vi "main.vi"() -> ()   [LabVIEW 2014]
uses:
  controls/addressPF.ctl
  controls/dataPF.ctl
  <vilib>/rvi/interface/nirviReadWriteControl/nirviReadWriteControl.xnode
  NiFpgaLv.dll
  <vilib>/Utility/error.llb/Error Cluster From Error Code.vi
  <vilib>/rvi/interface/Simulation/niFpgaSimulationCallBeginRW.vi
  <vilib>/rvi/errors/niLvFpgaAdjustHostInterfaceError.vi
  <vilib>/rvi/interface/nirviOpenFPGA/nirviOpenFPGA.xnode
  <vilib>/rvi/Analysis/host/Public/NI_FpgaMspHost.lvlib
  <vilib>/rvi/interface/nirviMethod/nirviMethod.xnode
  <vilib>/rvi/errors/niLvFpgaMergeErrorWithErrorCode.vi
  <vilib>/FPGAPlugInAG/Dynamic/niLvFpga_StartFifo_Dynamic.vi
  <vilib>/FPGAPlugInAG/Dynamic/niLvFpga_ConfigureFifo_Dynamic.vi
  <vilib>/FPGAPlugInAG/Dynamic/niLvFpga_ReadFifo_Dynamic.vi
  <vilib>/FPGAPlugInAG/Dynamic/niLvFpga_StopFifo_Dynamic.vi
  <vilib>/rvi/interface/nirviCloseFPGA/nirviCloseFPGA.xnode
  <vilib>/FPGAPlugInAG/Dynamic/niLvFpga_Close_Dynamic.vi
  <vilib>/FPGAPlugInAG/Dynamic/niLvFpga_Run_Dynamic.vi
  <vilib>/rvi/Analysis/host/Private/Sample Rate To Loop Time (ticks).vi
  FPGA Bitfiles/projetofinal_FPGATarget_acquiringdata_+swI5PFvCiE.lvbitx
  acquiring data.vi
  <vilib>/FPGAPlugInAG/myRIO-1900/niLvFpga_Open_myRIO-1900.vi
  <vilib>/rvi/interface/common/dynamic/niFpgaDynamicAddResources.vi
  FPGA Bitfiles/projetofinal_FPGATarget_fpga6_P5NV++MLsEc.lvbitx
  fpga6.vi
panel:
  out "Voltage":dbl[](array[numeric])
  out "Current":dbl[](array[numeric])
  in  "curvas":string(combo)
  out "Standart Deviation":dbl
  out "Mean":dbl
  in  "file name":string="measure"
  out "source":string
  out "status":bool
  out "code":i32
  in  "measure":bool
  in  "Wait":u32
  in  "acq":bool
  in  "save":bool
  out "contdown":i16
  in  "duration":dbl=5.0 format="%#_13g"
  in  "f (Hz)":dbl=50000.0 format="%#_6p"
  in  "Stop Button":bool
  out "FIFO full?":bool
  in  "set":bool
  in  "qvolt":i32
  in  "sens":i32
  in  "bi":bool
  in  "qvolt":bool
  in  "sens":bool caption="sensibility"
  in  "mode":string(combo)
  # "Programming"
  # "Acquisition"
  # "Save File"
  # "Sensibility"
  # "File Name"
  # "Frequency (Hz)"
  # "Quiescent Voltage"
  # "FIFO Full"
  # "Unipolar"
  # "Duration"
  # "Countdown"
  # "Measure"
  # "Wait"
  # "Error"
  # "Status"
  # "Source"
  # "Code"
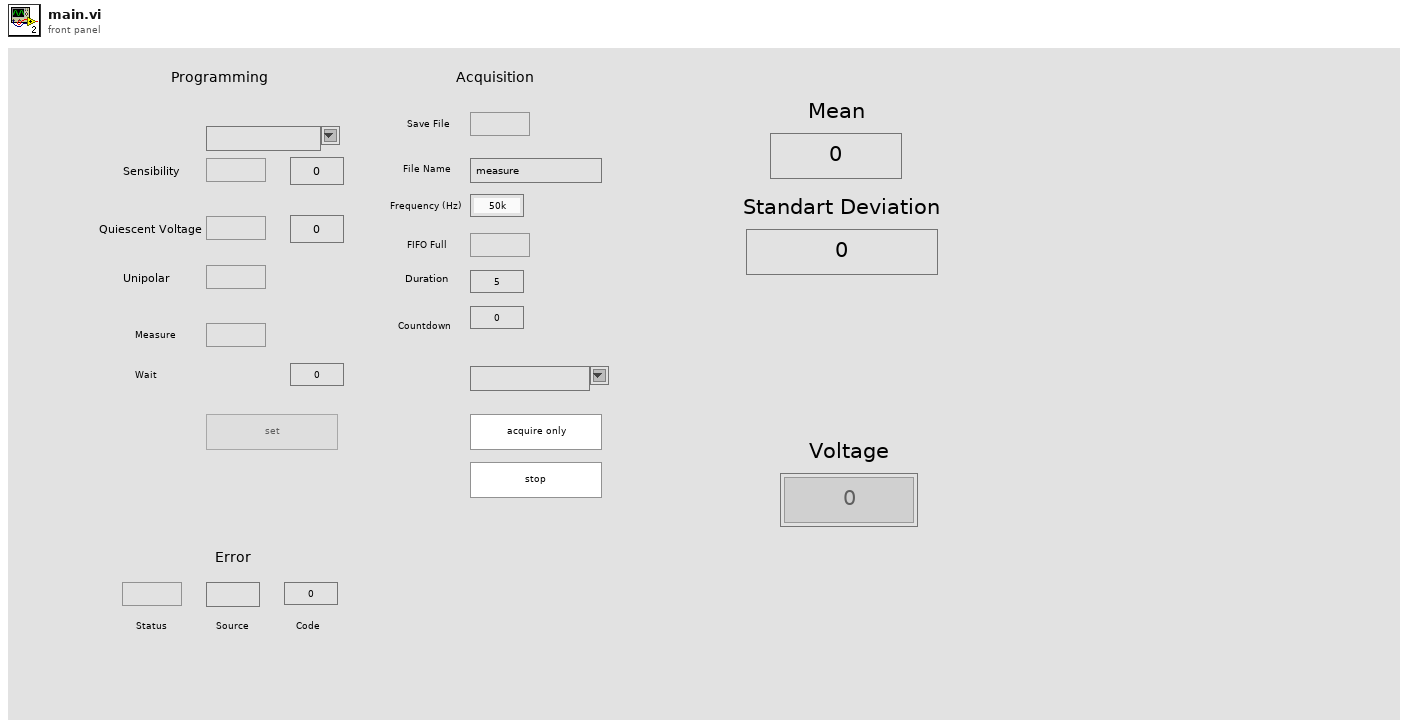
[diagram p1: front panel]
types:
  T1 = enum8{"Enabled", "Disabled", "Disabled and Grayed Out"}
  T2 = typedef "dataPF.ctl" = cluster{"sens":i32, "set?":bool, "mode":string, "parameters":cluster{"sens":bool, "qvolt":bool, "bi":bool}, "counter":i32, "qvolt":i32, "data":dbl[][], "fpga ref":refnum<k20>, "frequency":dbl}
  T3 = typedef "addressPF.ctl" = enum16{"idle", "lock", "set", "reset", "get data", "save data"}
  T4 = cluster{"mean":dbl, "standard deviation":dbl, "variance":dbl}
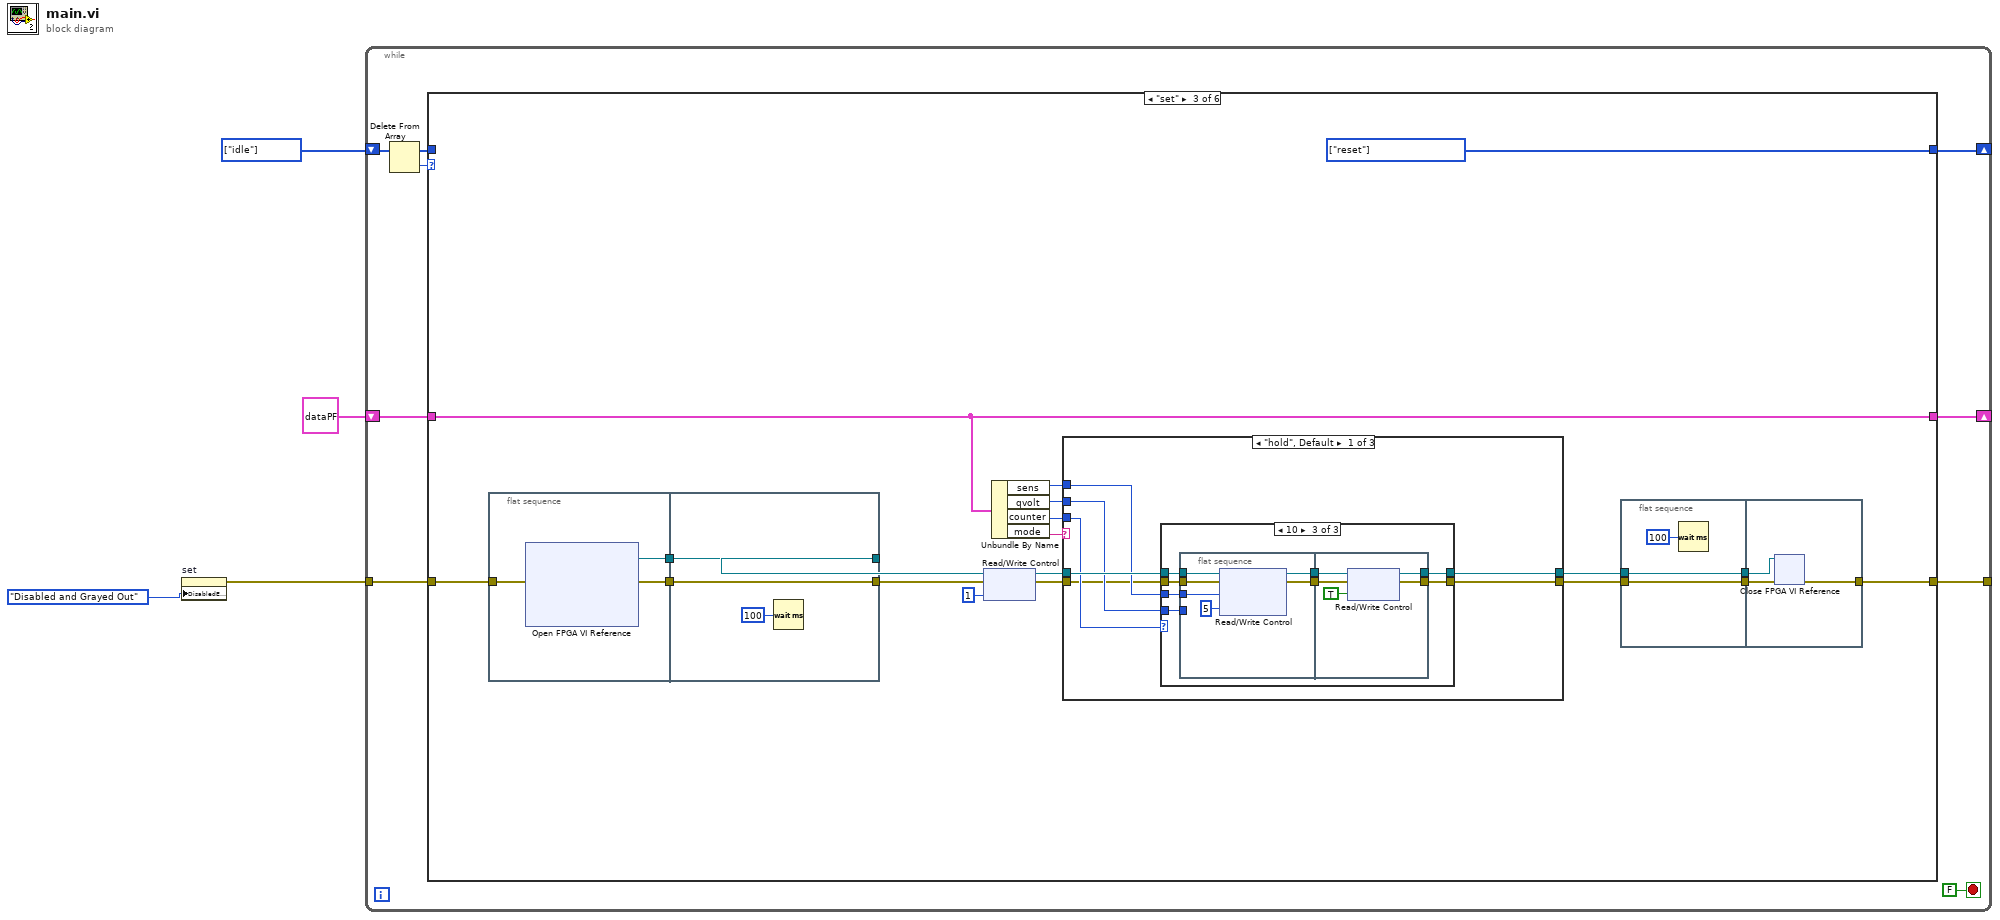
[diagram p0: block diagram]
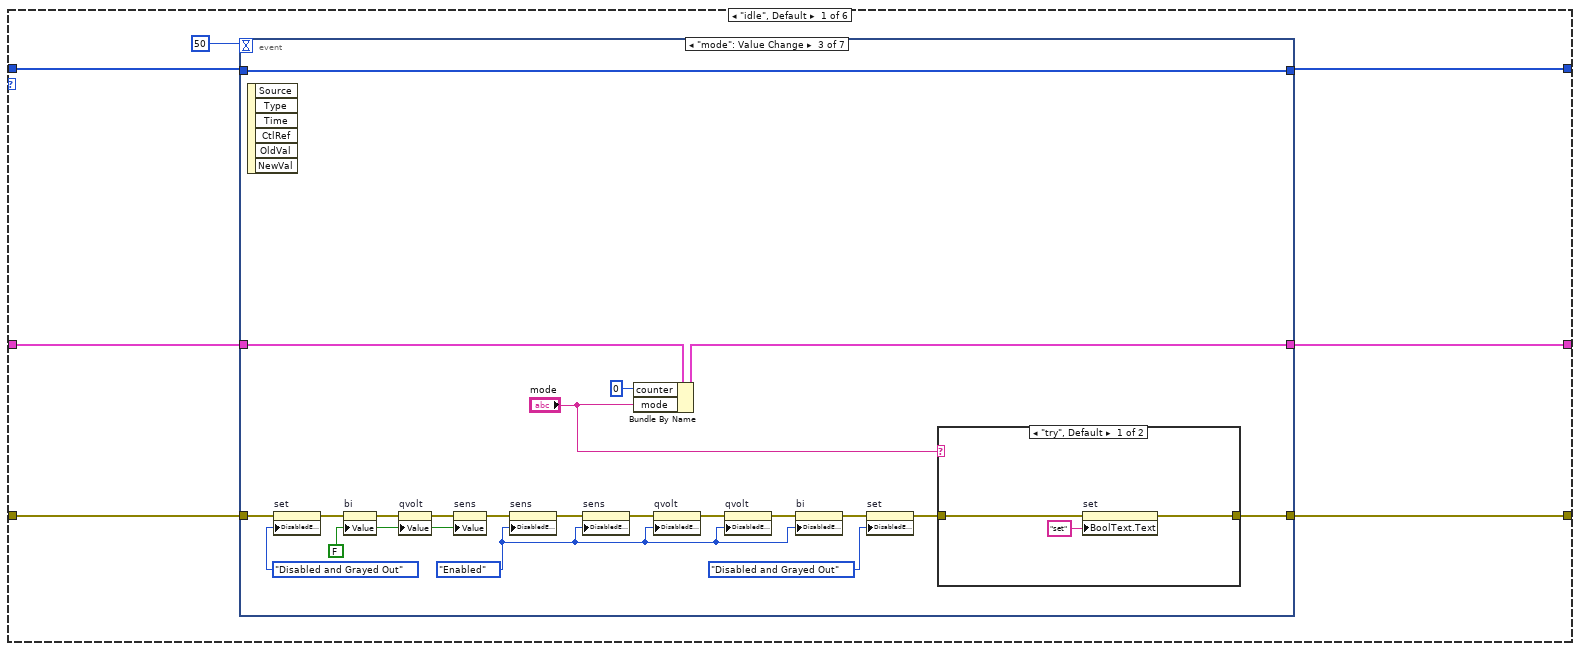
[diagram p2: hidden frame]
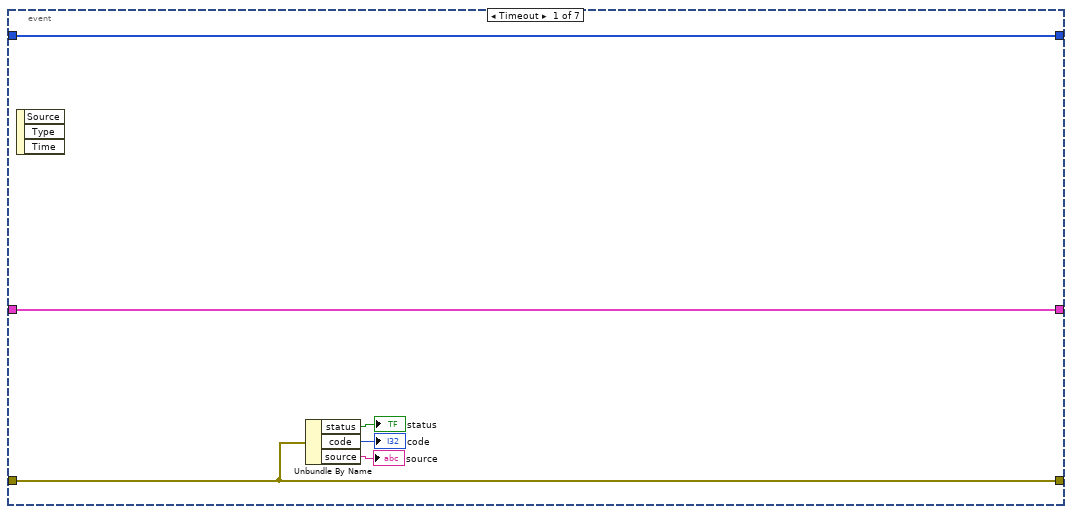
[diagram p3: hidden frame]
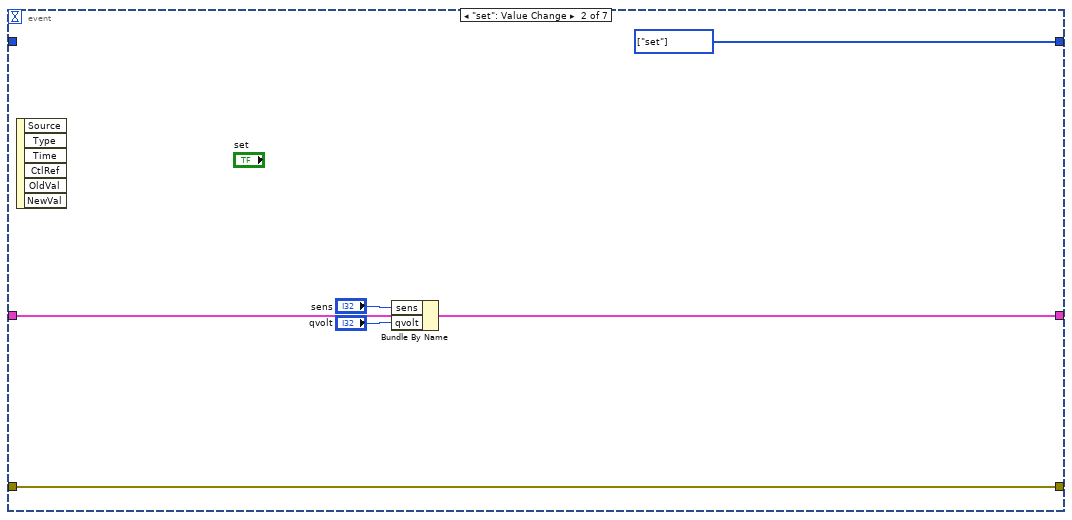
[diagram p4: hidden frame]
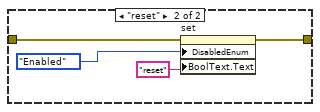
[diagram p5: hidden frame]
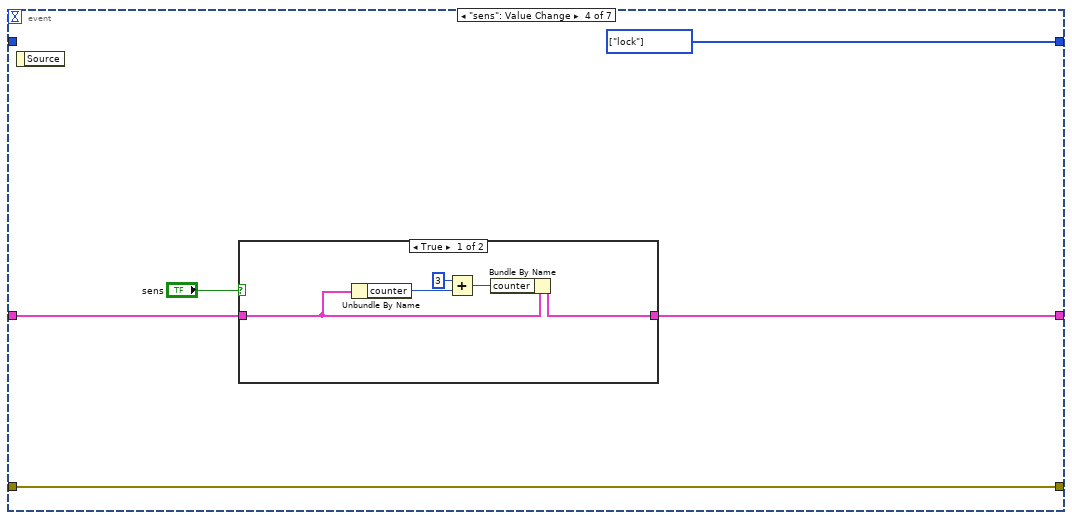
[diagram p6: hidden frame]
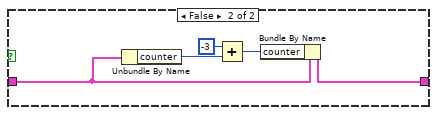
[diagram p7: hidden frame]
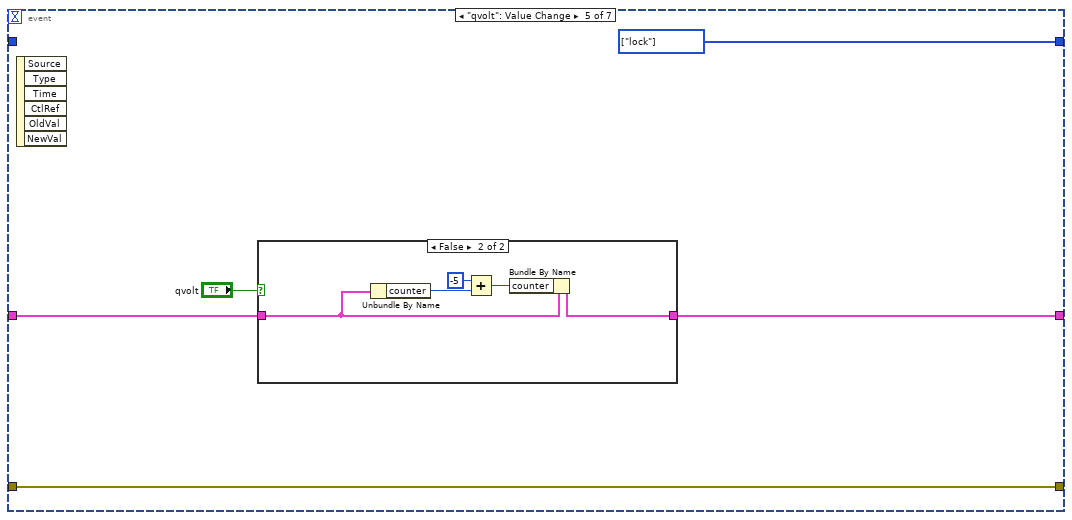
[diagram p8: hidden frame]
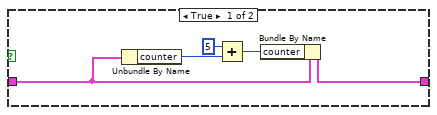
[diagram p9: hidden frame]
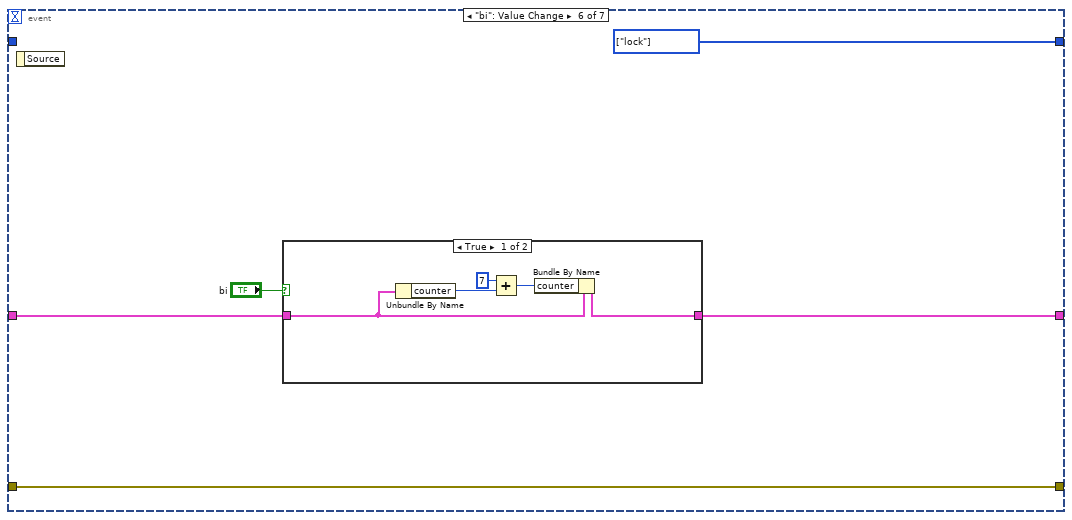
[diagram p10: hidden frame]
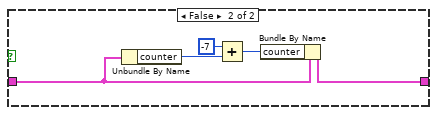
[diagram p11: hidden frame]
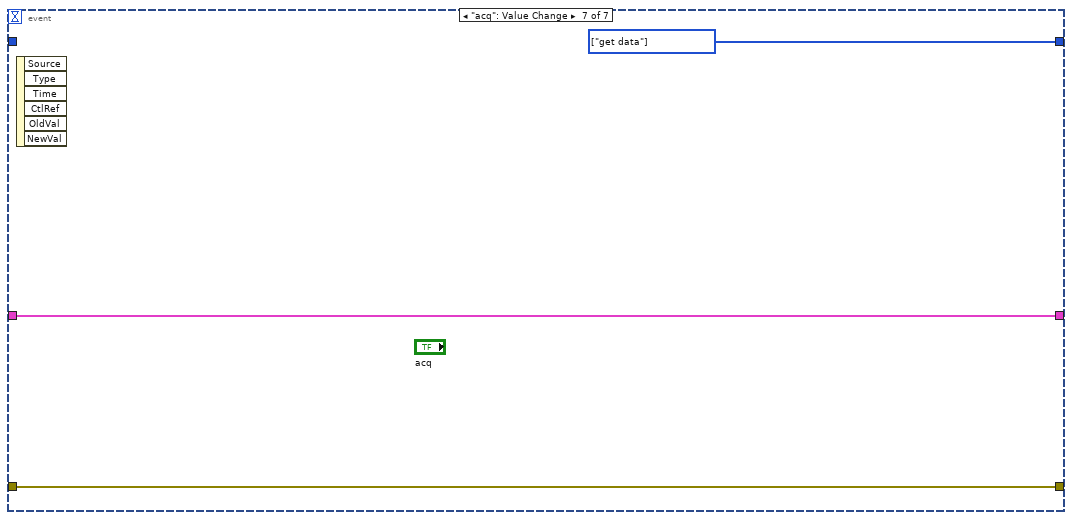
[diagram p12: hidden frame]
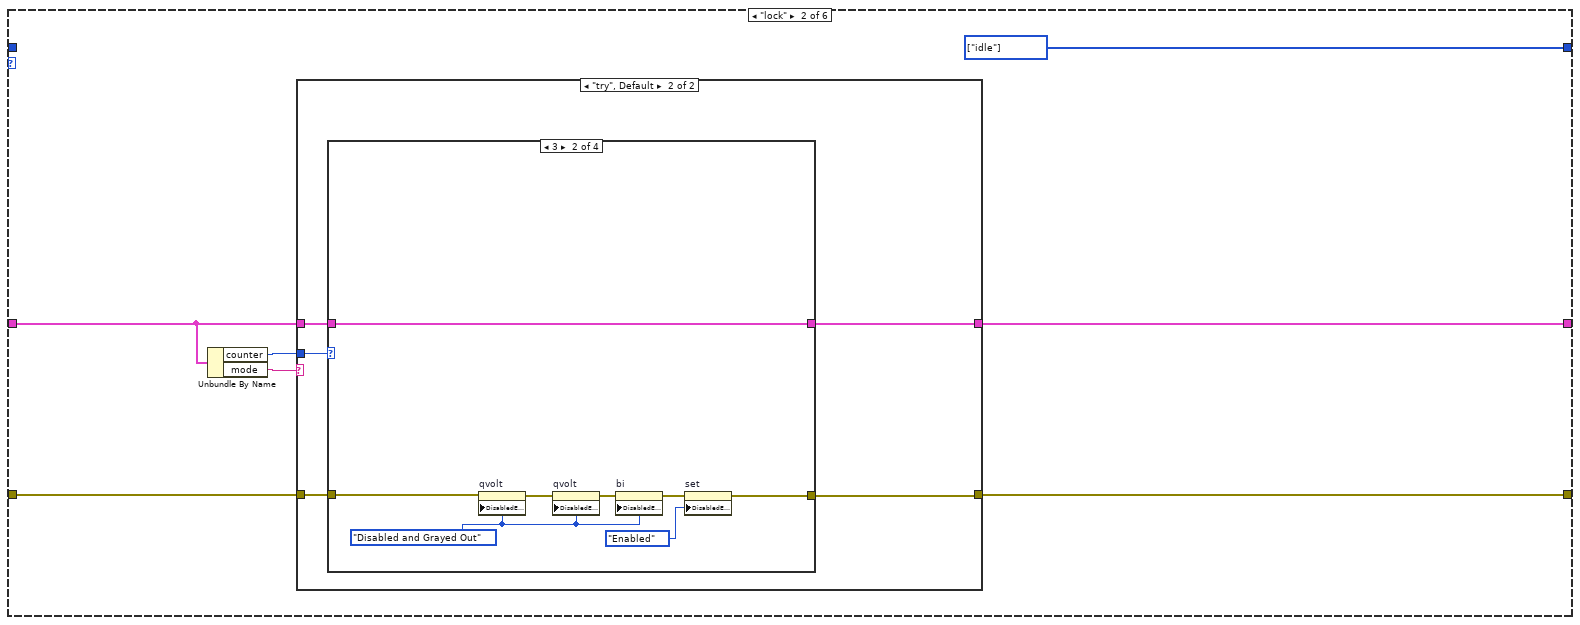
[diagram p13: hidden frame]
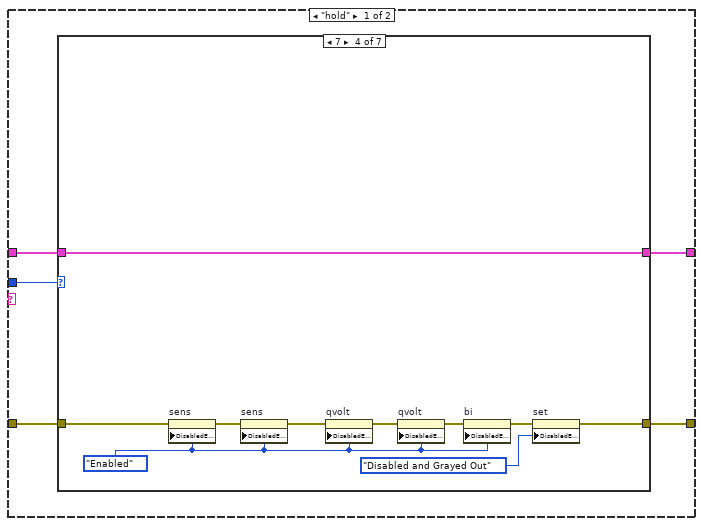
[diagram p14: hidden frame]
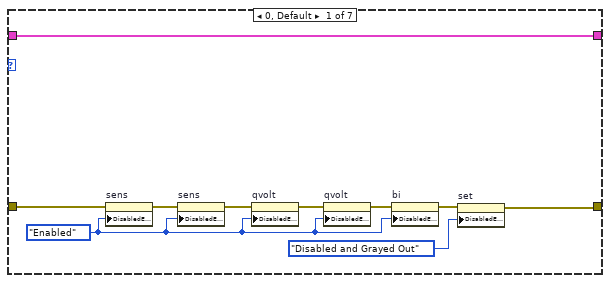
[diagram p15: hidden frame]
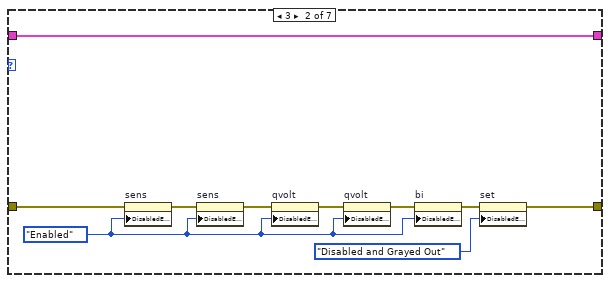
[diagram p16: hidden frame]
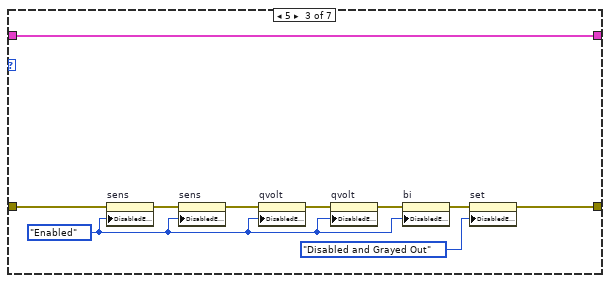
[diagram p17: hidden frame]
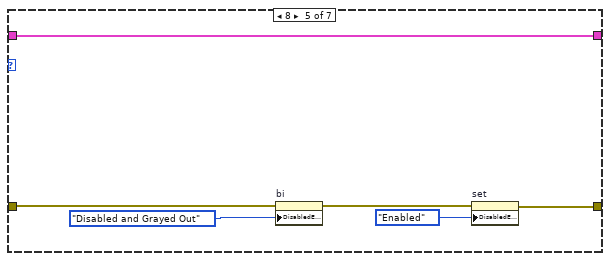
[diagram p18: hidden frame]
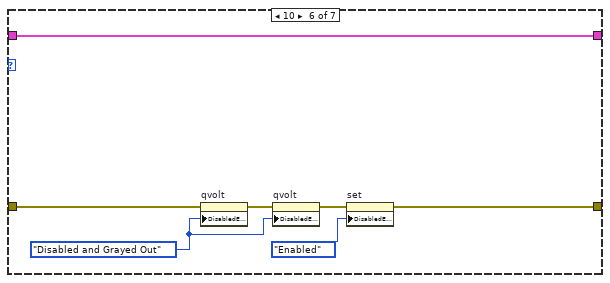
[diagram p19: hidden frame]
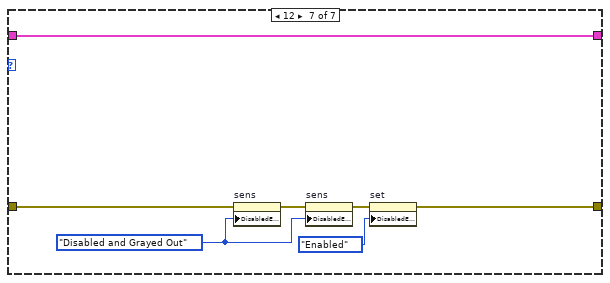
[diagram p20: hidden frame]
diagram:
  w4 = T3[] [enum."idle"] items=["idle", "lock", "set", "reset", "get data", "save data"]
  n1 = property on="set" class="Bool"("DisabledEnum"=T1."Disabled and Grayed Out" ("Disabled")) -> (error out=w1:errorcluster)  [unwired: 2 in, 1 out]
  n2 = while {
    shift-right: [w10] -> _
    shift-left: w4 -> [w13]
    shift-right: [w8] -> _
    shift-left: T2 {"sens"=0, "set?"=FALSE, "mode"="", "parameters"={"sens"=FALSE, "qvolt"=FALSE, "bi"=FALSE}, "counter"=0, "qvolt"=0, "data"=[], "fpga ref"=refnum, "frequency"=0.0} -> [w7]
    tunnel: w1 -> [w6]
    tunnel: [w5] -> _
    stop <- FALSE stop-if-true
    n3 = Delete From Array(array=w13) -> (deleted portion=w12:T3, array with subset deleted=w11:T3[])  [unwired: 2 in]
    n4 = case shown="\"set\"" w12 {
      tunnel: w11 -> [w20 _ _ _ _ _]
      tunnel: [w19 w115 w239 w384 w413 w493] -> w10
      tunnel: [w18 w112 w231 w386 w428 w492] -> w8
      tunnel: w7 -> [w17 w111 w231 w377 w430 w492]
      tunnel: w6 -> [w15 w110 w227 w380 w426 w485]
      tunnel: [w14 w109 w230 w385 w422 w490] -> w5
      frame "idle", Default {
        n5 = event shown="[2] \"mode\": Value Change" {
          selector: _ -> [_ _ _ _ _ _ _]
          dyn-events: _ -> [_ _ _ _ _ _ _]
          timeout: 50 -> [_ _ _ _ _ _ _]
          tunnel: w20 -> [w26 _ w53 _ _ _ _]
          tunnel: [w26 w32 w53 w65 w80 w95 w107] -> w19
          tunnel: [w25 w30 w51 w62 w79 w93 w106] -> w18
          tunnel: w17 -> [w25 w31 w52 w63 w78 w94 w106]
          tunnel: w15 -> [w24 w28 w37 w61 w76 w91 w108]
          tunnel: [w24 w28 w34 w61 w76 w91 w108] -> w14
          event Timeout {
            n6 = event-data() -> ()  [unwired: 1 in, 3 out]
            n7 = Unbundle By Name(w24) -> ("status"=→"status":bool, "code"=→"code":i32, "source"=→"source":string)
          }
          event "set": Value Change {
            w32 = T3[] [enum."set"] items=["idle", "lock", "set", "reset", "get data", "save data"]
            n8 = event-data() -> ()  [unwired: 1 in, 6 out]
            n9 = Bundle By Name(cluster=w31, "sens"="sens", "qvolt"="qvolt") -> (w30:T2)
          }
          event "mode": Value Change {
            w44 = T1."Enabled" ("Disabled")
            w50 = FALSE
            n10 = event-data() -> ()  [unwired: 1 in, 6 out]
            n11 = property on="set" class="Bool"(error in=w37, "DisabledEnum"=T1."Disabled and Grayed Out" ("Disabled")) -> (error out=w39:errorcluster)  [unwired: 1 in, 1 out]
            n12 = property on="bi" class="Bool (strict)"(error in=w39, "Value"=w50) -> (error out=w41:errorcluster)  [unwired: 1 in, 1 out]
            n13 = property on="qvolt" class="Bool (strict)"(error in=w41, "Value"=w50) -> (error out=w40:errorcluster)  [unwired: 1 in, 1 out]
            n14 = property on="sens" class="Bool (strict)"(error in=w40, "Value"=w50) -> (error out=w38:errorcluster)  [unwired: 1 in, 1 out]
            n15 = property on="sens" class="DigNum (strict)"(error in=w38, "DisabledEnum"=w44) -> (error out=w46:errorcluster)  [unwired: 1 in, 1 out]
            n16 = property on="sens" class="Bool (strict)"(error in=w46, "DisabledEnum"=w44) -> (error out=w36:errorcluster)  [unwired: 1 in, 1 out]
            n17 = Bundle By Name(cluster=w52, "counter"=0, "mode"="mode") -> (w51:T2)
            n18 = property on="qvolt" class="DigNum (strict)"(error in=w36, "DisabledEnum"=w44) -> (error out=w47:errorcluster)  [unwired: 1 in, 1 out]
            n19 = property on="qvolt" class="Bool (strict)"(error in=w47, "DisabledEnum"=w44) -> (error out=w48:errorcluster)  [unwired: 1 in, 1 out]
            n20 = property on="bi" class="Bool (strict)"(error in=w48, "DisabledEnum"=w44) -> (error out=w45:errorcluster)  [unwired: 1 in, 1 out]
            n21 = property on="set" class="Bool"(error in=w45, "DisabledEnum"=T1."Disabled and Grayed Out" ("Disabled")) -> (error out=w35:errorcluster)  [unwired: 1 in, 1 out]
            n22 = case shown="\"try\", Default" "mode" {
              tunnel: w35 -> [w56 w59]
              tunnel: [w55 w58] -> w34
              frame "try", Default {
                n23 = property on="set" class="Bool"(error in=w56, "BoolText.Text"="set" ("Boolean Text.Text")) -> (error out=w55:errorcluster)  [unwired: 1 in, 1 out]
              }
              frame "reset" {
                n24 = property on="set" class="Bool"(error in=w59, "DisabledEnum"=T1."Enabled" ("Disabled"), "BoolText.Text"="reset" ("Boolean Text.Text")) -> (error out=w58:errorcluster)  [unwired: 1 in, 1 out]
              }
            }
          }
          event "sens": Value Change {
            w65 = T3[] [enum."lock"] items=["idle", "lock", "set", "reset", "get data", "save data"]
            n25 = event-data() -> ()  [unwired: 1 in, 1 out]
            n26 = case shown="True" "sens" {
              tunnel: w63 -> [w67 w72]
              tunnel: [w66 w71] -> w62
              frame True {
                n27 = Unbundle By Name(w67) -> ("counter"=w69:i32)
                n28 = Add(x=3, y=w69) -> (x+y=w68:i32)
                n29 = Bundle By Name(cluster=w67, "counter"=w68) -> (w66:T2)
              }
              frame False {
                n30 = Unbundle By Name(w72) -> ("counter"=w74:i32)
                n31 = Add(x=-3, y=w74) -> (x+y=w73:i32)
                n32 = Bundle By Name(cluster=w72, "counter"=w73) -> (w71:T2)
              }
            }
          }
          event "qvolt": Value Change {
            w80 = T3[] [enum."lock"] items=["idle", "lock", "set", "reset", "get data", "save data"]
            n33 = event-data() -> ()  [unwired: 1 in, 6 out]
            n34 = case shown="False" "qvolt" {
              tunnel: w78 -> [w82 w87]
              tunnel: [w81 w86] -> w79
              frame True {
                n35 = Unbundle By Name(w82) -> ("counter"=w84:i32)
                n36 = Add(x=5, y=w84) -> (x+y=w83:i32)
                n37 = Bundle By Name(cluster=w82, "counter"=w83) -> (w81:T2)
              }
              frame False {
                n38 = Unbundle By Name(w87) -> ("counter"=w89:i32)
                n39 = Add(x=-5, y=w89) -> (x+y=w88:i32)
                n40 = Bundle By Name(cluster=w87, "counter"=w88) -> (w86:T2)
              }
            }
          }
          event "bi": Value Change {
            w95 = T3[] [enum."lock"] items=["idle", "lock", "set", "reset", "get data", "save data"]
            n41 = event-data() -> ()  [unwired: 1 in, 1 out]
            n42 = case shown="True" "bi" {
              tunnel: w94 -> [w97 w102]
              tunnel: [w96 w101] -> w93
              frame True {
                n43 = Unbundle By Name(w97) -> ("counter"=w99:i32)
                n44 = Add(x=7, y=w99) -> (x+y=w98:i32)
                n45 = Bundle By Name(cluster=w97, "counter"=w98) -> (w96:T2)
              }
              frame False {
                n46 = Unbundle By Name(w102) -> ("counter"=w104:i32)
                n47 = Add(x=-7, y=w104) -> (x+y=w103:i32)
                n48 = Bundle By Name(cluster=w102, "counter"=w103) -> (w101:T2)
              }
            }
          }
          event "acq": Value Change {
            w107 = T3[] [enum."get data"] items=["idle", "lock", "set", "reset", "get data", "save data"]
            n49 = event-data() -> ()  [unwired: 1 in, 6 out]
          }
        }
      }
      frame "lock" {
        w115 = T3[] [enum."idle"] items=["idle", "lock", "set", "reset", "get data", "save data"]
        n50 = Unbundle By Name(w111) -> ("counter"=w113:i32, "mode"=w114:string)
        n51 = case shown="\"try\", Default" w114 {
          tunnel: w113 -> [w120 w185]
          tunnel: [w116 w182] -> w112
          tunnel: w111 -> [w117 w181]
          tunnel: w110 -> [w119 w184]
          tunnel: [w118 w183] -> w109
          frame "hold" {
            n52 = case shown="7" w120 {
              tunnel: w119 -> [w124 w132 w144 w152 w162 w169 w176]
              tunnel: [w122 w133 w143 w153 w164 w168 w174] -> w118
              tunnel: w117 -> [w121 w131 w141 w151 w161 w167 w177]
              tunnel: [w121 w131 w141 w151 w161 w167 w177] -> w116
              frame 0, Default {
                w126 = T1."Enabled" ("Disabled")
                n53 = property on="sens" class="DigNum (strict)"(error in=w124, "DisabledEnum"=w126) -> (error out=w127:errorcluster)  [unwired: 1 in, 1 out]
                n54 = property on="sens" class="Bool (strict)"(error in=w127, "DisabledEnum"=w126) -> (error out=w128:errorcluster)  [unwired: 1 in, 1 out]
                n55 = property on="qvolt" class="DigNum (strict)"(error in=w128, "DisabledEnum"=w126) -> (error out=w129:errorcluster)  [unwired: 1 in, 1 out]
                n56 = property on="qvolt" class="Bool (strict)"(error in=w129, "DisabledEnum"=w126) -> (error out=w130:errorcluster)  [unwired: 1 in, 1 out]
                n57 = property on="bi" class="Bool (strict)"(error in=w130, "DisabledEnum"=w126) -> (error out=w123:errorcluster)  [unwired: 1 in, 1 out]
                n58 = property on="set" class="Bool"(error in=w123, "DisabledEnum"=T1."Disabled and Grayed Out" ("Disabled")) -> (error out=w122:errorcluster)  [unwired: 1 in, 1 out]
              }
              frame 3 {
                w136 = T1."Enabled" ("Disabled")
                n59 = property on="sens" class="DigNum (strict)"(error in=w132, "DisabledEnum"=w136) -> (error out=w137:errorcluster)  [unwired: 1 in, 1 out]
                n60 = property on="sens" class="Bool (strict)"(error in=w137, "DisabledEnum"=w136) -> (error out=w138:errorcluster)  [unwired: 1 in, 1 out]
                n61 = property on="qvolt" class="DigNum (strict)"(error in=w138, "DisabledEnum"=w136) -> (error out=w139:errorcluster)  [unwired: 1 in, 1 out]
                n62 = property on="qvolt" class="Bool (strict)"(error in=w139, "DisabledEnum"=w136) -> (error out=w140:errorcluster)  [unwired: 1 in, 1 out]
                n63 = property on="bi" class="Bool (strict)"(error in=w140, "DisabledEnum"=w136) -> (error out=w134:errorcluster)  [unwired: 1 in, 1 out]
                n64 = property on="set" class="Bool"(error in=w134, "DisabledEnum"=T1."Disabled and Grayed Out" ("Disabled")) -> (error out=w133:errorcluster)  [unwired: 1 in, 1 out]
              }
              frame 5 {
                w142 = T1."Enabled" ("Disabled")
                n65 = property on="sens" class="DigNum (strict)"(error in=w144, "DisabledEnum"=w142) -> (error out=w147:errorcluster)  [unwired: 1 in, 1 out]
                n66 = property on="sens" class="Bool (strict)"(error in=w147, "DisabledEnum"=w142) -> (error out=w148:errorcluster)  [unwired: 1 in, 1 out]
                n67 = property on="qvolt" class="DigNum (strict)"(error in=w148, "DisabledEnum"=w142) -> (error out=w149:errorcluster)  [unwired: 1 in, 1 out]
                n68 = property on="qvolt" class="Bool (strict)"(error in=w149, "DisabledEnum"=w142) -> (error out=w150:errorcluster)  [unwired: 1 in, 1 out]
                n69 = property on="bi" class="Bool (strict)"(error in=w150, "DisabledEnum"=w142) -> (error out=w145:errorcluster)  [unwired: 1 in, 1 out]
                n70 = property on="set" class="Bool"(error in=w145, "DisabledEnum"=T1."Disabled and Grayed Out" ("Disabled")) -> (error out=w143:errorcluster)  [unwired: 1 in, 1 out]
              }
              frame 7 {
                w156 = T1."Enabled" ("Disabled")
                n71 = property on="sens" class="DigNum (strict)"(error in=w152, "DisabledEnum"=w156) -> (error out=w157:errorcluster)  [unwired: 1 in, 1 out]
                n72 = property on="sens" class="Bool (strict)"(error in=w157, "DisabledEnum"=w156) -> (error out=w158:errorcluster)  [unwired: 1 in, 1 out]
                n73 = property on="qvolt" class="DigNum (strict)"(error in=w158, "DisabledEnum"=w156) -> (error out=w159:errorcluster)  [unwired: 1 in, 1 out]
                n74 = property on="qvolt" class="Bool (strict)"(error in=w159, "DisabledEnum"=w156) -> (error out=w160:errorcluster)  [unwired: 1 in, 1 out]
                n75 = property on="bi" class="Bool (strict)"(error in=w160, "DisabledEnum"=w156) -> (error out=w154:errorcluster)  [unwired: 1 in, 1 out]
                n76 = property on="set" class="Bool"(error in=w154, "DisabledEnum"=T1."Disabled and Grayed Out" ("Disabled")) -> (error out=w153:errorcluster)  [unwired: 1 in, 1 out]
              }
              frame 8 {
                n77 = property on="bi" class="Bool (strict)"(error in=w162, "DisabledEnum"=T1."Disabled and Grayed Out" ("Disabled")) -> (error out=w163:errorcluster)  [unwired: 1 in, 1 out]
                n78 = property on="set" class="Bool"(error in=w163, "DisabledEnum"=T1."Enabled" ("Disabled")) -> (error out=w164:errorcluster)  [unwired: 1 in, 1 out]
              }
              frame 10 {
                w172 = T1."Disabled and Grayed Out" ("Disabled")
                n79 = property on="qvolt" class="DigNum (strict)"(error in=w169, "DisabledEnum"=w172) -> (error out=w173:errorcluster)  [unwired: 1 in, 1 out]
                n80 = property on="qvolt" class="Bool (strict)"(error in=w173, "DisabledEnum"=w172) -> (error out=w170:errorcluster)  [unwired: 1 in, 1 out]
                n81 = property on="set" class="Bool"(error in=w170, "DisabledEnum"=T1."Enabled" ("Disabled")) -> (error out=w168:errorcluster)  [unwired: 1 in, 1 out]
              }
              frame 12 {
                w179 = T1."Disabled and Grayed Out" ("Disabled")
                n82 = property on="sens" class="DigNum (strict)"(error in=w176, "DisabledEnum"=w179) -> (error out=w180:errorcluster)  [unwired: 1 in, 1 out]
                n83 = property on="sens" class="Bool (strict)"(error in=w180, "DisabledEnum"=w179) -> (error out=w175:errorcluster)  [unwired: 1 in, 1 out]
                n84 = property on="set" class="Bool"(error in=w175, "DisabledEnum"=T1."Enabled" ("Disabled")) -> (error out=w174:errorcluster)  [unwired: 1 in, 1 out]
              }
            }
          }
          frame "try", Default {
            n85 = case shown="3" w185 {
              tunnel: w184 -> [w187 w199 w205 w213]
              tunnel: [w188 w198 w206 w214] -> w183
              tunnel: [w186 w196 w204 w212] -> w182
              tunnel: w181 -> [w186 w196 w204 w212]
              frame 0, Default {
                w190 = T1."Enabled" ("Disabled")
                n86 = property on="sens" class="DigNum (strict)"(error in=w187, "DisabledEnum"=w190) -> (error out=w192:errorcluster)  [unwired: 1 in, 1 out]
                n87 = property on="sens" class="Bool (strict)"(error in=w192, "DisabledEnum"=w190) -> (error out=w193:errorcluster)  [unwired: 1 in, 1 out]
                n88 = property on="qvolt" class="DigNum (strict)"(error in=w193, "DisabledEnum"=w190) -> (error out=w194:errorcluster)  [unwired: 1 in, 1 out]
                n89 = property on="qvolt" class="Bool (strict)"(error in=w194, "DisabledEnum"=w190) -> (error out=w195:errorcluster)  [unwired: 1 in, 1 out]
                n90 = property on="bi" class="Bool (strict)"(error in=w195, "DisabledEnum"=w190) -> (error out=w191:errorcluster)  [unwired: 1 in, 1 out]
                n91 = property on="set" class="Bool"(error in=w191, "DisabledEnum"=T1."Disabled and Grayed Out" ("Disabled")) -> (error out=w188:errorcluster)  [unwired: 1 in, 1 out]
              }
              frame 3 {
                w197 = T1."Disabled and Grayed Out" ("Disabled")
                n92 = property on="qvolt" class="DigNum (strict)"(error in=w199, "DisabledEnum"=w197) -> (error out=w202:errorcluster)  [unwired: 1 in, 1 out]
                n93 = property on="qvolt" class="Bool (strict)"(error in=w202, "DisabledEnum"=w197) -> (error out=w203:errorcluster)  [unwired: 1 in, 1 out]
                n94 = property on="bi" class="Bool (strict)"(error in=w203, "DisabledEnum"=w197) -> (error out=w201:errorcluster)  [unwired: 1 in, 1 out]
                n95 = property on="set" class="Bool"(error in=w201, "DisabledEnum"=T1."Enabled" ("Disabled")) -> (error out=w198:errorcluster)  [unwired: 1 in, 1 out]
              }
              frame 5 {
                w210 = T1."Disabled and Grayed Out" ("Disabled")
                n96 = property on="sens" class="DigNum (strict)"(error in=w205, "DisabledEnum"=w210) -> (error out=w211:errorcluster)  [unwired: 1 in, 1 out]
                n97 = property on="sens" class="Bool (strict)"(error in=w211, "DisabledEnum"=w210) -> (error out=w209:errorcluster)  [unwired: 1 in, 1 out]
                n98 = property on="bi" class="Bool (strict)"(error in=w209, "DisabledEnum"=w210) -> (error out=w208:errorcluster)  [unwired: 1 in, 1 out]
                n99 = property on="set" class="Bool"(error in=w208, "DisabledEnum"=T1."Enabled" ("Disabled")) -> (error out=w206:errorcluster)  [unwired: 1 in, 1 out]
              }
              frame 7 {
                w218 = T1."Disabled and Grayed Out" ("Disabled")
                n100 = property on="sens" class="DigNum (strict)"(error in=w213, "DisabledEnum"=w218) -> (error out=w219:errorcluster)  [unwired: 1 in, 1 out]
                n101 = property on="sens" class="Bool (strict)"(error in=w219, "DisabledEnum"=w218) -> (error out=w217:errorcluster)  [unwired: 1 in, 1 out]
                n102 = property on="qvolt" class="DigNum (strict)"(error in=w217, "DisabledEnum"=w218) -> (error out=w220:errorcluster)  [unwired: 1 in, 1 out]
                n103 = property on="qvolt" class="Bool (strict)"(error in=w220, "DisabledEnum"=w218) -> (error out=w216:errorcluster)  [unwired: 1 in, 1 out]
                n104 = property on="set" class="Bool"(error in=w216, "DisabledEnum"=T1."Enabled" ("Disabled")) -> (error out=w214:errorcluster)  [unwired: 1 in, 1 out]
              }
            }
          }
        }
      }
      frame "set" {
        w239 = T3[] [enum."reset"] items=["idle", "lock", "set", "reset", "get data", "save data"]
        n105 = flat-sequence {
          tunnel: w227 -> [w242]
          tunnel: [w241] -> w222
          tunnel: [w240] -> w221
          tunnel: [w244] -> w225
          tunnel: [w245] -> w226
          tunnel: w222 -> [w245]
          tunnel: w221 -> [w244]
          frame #0 {
            n106 = xnode "Open FPGA VI Reference"("error in"=w242) -> ("FPGA VI Reference Out"=w240:refnum<k20>, "error out"=w241:errorcluster)  [unwired: 1 in]
          }
          frame #1 {
            n107 = Wait (ms)(milliseconds to wait=u32 100) -> ()  [unwired: 1 out]
          }
        }
        n108 = xnode "Read/Write Control"("FPGA VI Reference In"=w225, "error in"=w226, "treset"=u32 1) -> ("FPGA VI Reference Out"=w234:refnum<k20>, "error out"=w232:errorcluster)
        n109 = Unbundle By Name(w231) -> ("sens"=w236:i32, "qvolt"=w235:i32, "counter"=w237:i32, "mode"=w238:string)
        n110 = case shown="\"hold\", Default" w238 {
          tunnel: w237 -> [w257 _ w322]
          tunnel: w234 -> [w258 w303 w321]
          tunnel: w236 -> [w256 _ w320]
          tunnel: w235 -> [w255 _ w319]
          tunnel: [w254 w301 w318] -> w228
          tunnel: [w253 w300 w316] -> w229
          tunnel: w232 -> [w252 w302 w317]
          frame "hold", Default {
            n111 = case shown="10" w257 {
              tunnel: w258 -> [w260 w268 w288]
              tunnel: w256 -> [_ w267 w287]
              tunnel: w255 -> [_ w266 w286]
              tunnel: [w260 w264 w284] -> w254
              tunnel: [w259 w261 w281] -> w253
              tunnel: w252 -> [w259 w263 w283]
              frame 0, Default {
              }
              frame 8 {
                n112 = flat-sequence {
                  tunnel: w268 -> [w275]
                  tunnel: w267 -> [w274]
                  tunnel: w266 -> [w273]
                  tunnel: [w271] -> w265
                  tunnel: w263 -> [w270]
                  tunnel: [w269] -> w262
                  tunnel: w265 -> [w280]
                  tunnel: [w278] -> w264
                  tunnel: w262 -> [w277]
                  tunnel: [w276] -> w261
                  frame #0 {
                    n113 = xnode "Read/Write Control"("FPGA VI Reference In"=w275, "error in"=w270, "hsens1"=w274, "hqvolt1"=w273, "parameter"=i16 4) -> ("FPGA VI Reference Out"=w271:refnum<k20>, "error out"=w269:errorcluster)
                  }
                  frame #1 {
                    n114 = xnode "Read/Write Control"("FPGA VI Reference In"=w280, "error in"=w277, "set"=TRUE) -> ("FPGA VI Reference Out"=w278:refnum<k20>, "error out"=w276:errorcluster)
                  }
                }
              }
              frame 10 {
                n115 = flat-sequence {
                  tunnel: w288 -> [w294]
                  tunnel: w287 -> [w293]
                  tunnel: w286 -> [_]
                  tunnel: [w291] -> w285
                  tunnel: w283 -> [w290]
                  tunnel: [w289] -> w282
                  tunnel: w285 -> [w299]
                  tunnel: [w297] -> w284
                  tunnel: w282 -> [w296]
                  tunnel: [w295] -> w281
                  frame #0 {
                    n116 = xnode "Read/Write Control"("FPGA VI Reference In"=w294, "error in"=w290, "hsens2"=w293, "parameter"=i16 5) -> ("FPGA VI Reference Out"=w291:refnum<k20>, "error out"=w289:errorcluster)
                  }
                  frame #1 {
                    n117 = xnode "Read/Write Control"("FPGA VI Reference In"=w299, "error in"=w296, "set"=TRUE) -> ("FPGA VI Reference Out"=w297:refnum<k20>, "error out"=w295:errorcluster)
                  }
                }
              }
            }
          }
          frame "reset" {
            n118 = flat-sequence {
              tunnel: w302 -> [w309]
              tunnel: [w308] -> w305
              tunnel: [w307] -> w304
              tunnel: w303 -> [w306]
              tunnel: [w314] -> w301
              tunnel: w305 -> [w313]
              tunnel: [w312] -> w300
              tunnel: w304 -> [w311]
              frame #0 {
                n119 = xnode "Read/Write Control"("FPGA VI Reference In"=w306, "error in"=w309, "parameter"=i16 6) -> ("FPGA VI Reference Out"=w307:refnum<k20>, "error out"=w308:errorcluster)
              }
              frame #1 {
                n120 = xnode "Read/Write Control"("FPGA VI Reference In"=w311, "error in"=w313, "set"=TRUE) -> ("FPGA VI Reference Out"=w314:refnum<k20>, "error out"=w312:errorcluster)
              }
            }
          }
          frame "try" {
            n121 = case shown="3" w322 {
              tunnel: w321 -> [w324 w325 w349 w366]
              tunnel: w320 -> [_ w331 _ _]
              tunnel: w319 -> [_ _ w347 _]
              tunnel: [w324 w330 w346 w364] -> w318
              tunnel: w317 -> [w323 w329 w345 w363]
              tunnel: [w323 w327 w343 w361] -> w316
              frame 0, Default {
              }
              frame 3 {
                n122 = flat-sequence {
                  tunnel: w331 -> [w337]
                  tunnel: w329 -> [w335]
                  tunnel: [w334] -> w328
                  tunnel: [w333] -> w326
                  tunnel: w325 -> [w332]
                  tunnel: [w341] -> w330
                  tunnel: w328 -> [w340]
                  tunnel: [w339] -> w327
                  tunnel: w326 -> [w338]
                  frame #0 {
                    n123 = xnode "Read/Write Control"("FPGA VI Reference In"=w332, "error in"=w335, "sens"=w337, "parameter"=i16 1) -> ("FPGA VI Reference Out"=w333:refnum<k20>, "error out"=w334:errorcluster)
                  }
                  frame #1 {
                    n124 = xnode "Read/Write Control"("FPGA VI Reference In"=w338, "error in"=w340, "set"=TRUE) -> ("FPGA VI Reference Out"=w341:refnum<k20>, "error out"=w339:errorcluster)
                  }
                }
              }
              frame 5 {
                n125 = flat-sequence {
                  tunnel: w349 -> [w355]
                  tunnel: [w354] -> w348
                  tunnel: w347 -> [w352]
                  tunnel: w345 -> [w351]
                  tunnel: [w350] -> w344
                  tunnel: w348 -> [w359]
                  tunnel: [w358] -> w346
                  tunnel: w344 -> [w357]
                  tunnel: [w356] -> w343
                  frame #0 {
                    n126 = xnode "Read/Write Control"("FPGA VI Reference In"=w355, "error in"=w351, "qv"=w352, "parameter"=i16 2) -> ("FPGA VI Reference Out"=w354:refnum<k20>, "error out"=w350:errorcluster)
                  }
                  frame #1 {
                    n127 = xnode "Read/Write Control"("FPGA VI Reference In"=w359, "error in"=w357, "set"=TRUE) -> ("FPGA VI Reference Out"=w358:refnum<k20>, "error out"=w356:errorcluster)
                  }
                }
              }
              frame 7 {
                n128 = flat-sequence {
                  tunnel: w366 -> [w371]
                  tunnel: [w370] -> w365
                  tunnel: w363 -> [w368]
                  tunnel: [w367] -> w362
                  tunnel: w365 -> [w375]
                  tunnel: [w374] -> w364
                  tunnel: w362 -> [w373]
                  tunnel: [w372] -> w361
                  frame #0 {
                    n129 = xnode "Read/Write Control"("FPGA VI Reference In"=w371, "error in"=w368, "parameter"=i16 3) -> ("FPGA VI Reference Out"=w370:refnum<k20>, "error out"=w367:errorcluster)
                  }
                  frame #1 {
                    n130 = xnode "Read/Write Control"("FPGA VI Reference In"=w375, "error in"=w373, "set"=TRUE) -> ("FPGA VI Reference Out"=w374:refnum<k20>, "error out"=w372:errorcluster)
                  }
                }
              }
            }
          }
        }
        n131 = flat-sequence {
          tunnel: w228 -> [w247]
          tunnel: w229 -> [w248]
          tunnel: [w248] -> w224
          tunnel: [w247] -> w223
          tunnel: [w251] -> w230
          tunnel: w224 -> [w250]
          tunnel: w223 -> [w249]
          frame #0 {
            n132 = Wait (ms)(milliseconds to wait=u32 100) -> ()  [unwired: 1 out]
          }
          frame #1 {
            n133 = xnode "Close FPGA VI Reference"("FPGA VI Reference In"=w249, "error in"=w250) -> ("error out"=w251:errorcluster)
          }
        }
      }
      frame "reset" {
        w381 = T3[] [enum."idle"] items=["idle", "lock", "set", "reset", "get data", "save data"]
        w383 = T3[] [enum."get data"] items=["idle", "lock", "set", "reset", "get data", "save data"]
        n134 = flat-sequence {
          tunnel: [w390] -> w379
          tunnel: [w387] -> w378
          tunnel: w380 -> [w389]
          tunnel: w377 -> [w388]
          tunnel: [w410] -> w385
          tunnel: [w411] -> w386
          tunnel: w379 -> [w411]
          tunnel: w378 -> [w410]
          frame #0 {
            w397 = T1."Enabled" ("Disabled")
            w404 = FALSE
            n135 = property on="bi" class="Bool (strict)"(error in=w389, "Value"=w404) -> (error out=w394:errorcluster)  [unwired: 1 in, 1 out]
            n136 = property on="qvolt" class="Bool (strict)"(error in=w394, "Value"=w404) -> (error out=w393:errorcluster)  [unwired: 1 in, 1 out]
            n137 = property on="sens" class="Bool (strict)"(error in=w393, "Value"=w404) -> (error out=w392:errorcluster)  [unwired: 1 in, 1 out]
            n138 = property on="sens" class="DigNum (strict)"(error in=w392, "DisabledEnum"=w397) -> (error out=w399:errorcluster)  [unwired: 1 in, 1 out]
            n139 = property on="sens" class="Bool (strict)"(error in=w399, "DisabledEnum"=w397) -> (error out=w400:errorcluster)  [unwired: 1 in, 1 out]
            n140 = property on="qvolt" class="DigNum (strict)"(error in=w400, "DisabledEnum"=w397) -> (error out=w401:errorcluster)  [unwired: 1 in, 1 out]
            n141 = property on="qvolt" class="Bool (strict)"(error in=w401, "DisabledEnum"=w397) -> (error out=w402:errorcluster)  [unwired: 1 in, 1 out]
            n142 = property on="bi" class="Bool (strict)"(error in=w402, "DisabledEnum"=w397) -> (error out=w398:errorcluster)  [unwired: 1 in, 1 out]
            n143 = Bundle By Name(cluster=w388, "counter"=0) -> (w390:T2)
            n144 = property on="set" class="Bool"(error in=w398, "DisabledEnum"=T1."Disabled and Grayed Out" ("Disabled")) -> (error out=w391:errorcluster)  [unwired: 1 in, 1 out]
            n145 = property on="set" class="Bool"(error in=w391, "DisabledEnum"=T1."Disabled and Grayed Out" ("Disabled")) -> (error out=w387:errorcluster)  [unwired: 1 in, 1 out]
          }
          frame #1 {
            n146 = To Double Precision Float(number="Wait") -> (double precision float=w406:dbl)
            n147 = Multiply(x=w406, y=1000.0) -> (x*y=w408:dbl)
            n148 = To Unsigned Long Integer(number=w408) -> (unsigned 32bit integer=w409:u32)
            n149 = Wait (ms)(milliseconds to wait=w409) -> ()  [unwired: 1 out]
          }
        }
        n150 = Select(t=w383, s="measure", f=w381) -> (s? t:f=w384:T3[])
      }
      frame "get data" {
        w414 = T3[] [enum."idle"] items=["idle", "lock", "set", "reset", "get data", "save data"]
        w416 = T3[] [enum."save data"] items=["idle", "lock", "set", "reset", "get data", "save data"]
        n151 = xnode "Open FPGA VI Reference"("error in"=w426) -> ("FPGA VI Reference Out"=w427:refnum<k20>, "error out"=w425:errorcluster)  [unwired: 1 in]
        n152 = xnode "Invoke Method"("FPGA VI Reference In"=w427, "error in"=w425) -> ("FPGA VI Reference Out"=w433:refnum<k20>, "error out"=w432:errorcluster)
        n153 = xnode "Invoke Method"("FPGA VI Reference In"=w433, "error in"=w432, "Requested Depth"=u32 10000) -> ("FPGA VI Reference Out"=w421:refnum<k20>, "error out"=w418:errorcluster)  [unwired: 1 out]
        n154 = xnode "Invoke Method"("FPGA VI Reference In"=w421, "error in"=w418, "Wait Until Done (F)"=FALSE) -> ("FPGA VI Reference Out"=w420:refnum<k20>, "error out"=w419:errorcluster)
        n155 = flat-sequence {
          tunnel: [w443] -> w435
          tunnel: [w442] -> w434
          tunnel: [w439] -> w429
          tunnel: w420 -> [w438]
          tunnel: w419 -> [w437]
          tunnel: [w436] -> w412
          frame #0 {
            n156 = Get Date/Time In Seconds() -> (seconds since 1Jan1904=w441:timestamp)
            n157 = while {
              shift-right: [w455] -> w442
              shift-left: w437 -> [w476]
              shift-right: [w460] -> w439
              shift-left: dbl[][] [] -> [w461]
              tunnel: w441 -> [w463]
              tunnel: [w454] -> w443
              tunnel: w438 -> [w459]
              tunnel: ["f (Hz)"] -> w436
              stop <- w471 stop-if-true
              # "Read Data"
              n158 = Get Date/Time In Seconds() -> (seconds since 1Jan1904=w464:timestamp)
              n159 = Subtract(x=w464, y=w463) -> (x-y=w452:dbl)
              n160 = call-poly <vilib>:"Sample Rate To Loop Time.vi"("sample rate (S/s)"="f (Hz)", "FPGA clock rate (Hz)"=40000000.0, "error in (no error)"=w476) -> ("count (ticks/S)"=w474:u32, "error out"=w469:errorcluster)  [unwired: 10 in, 1 out]
              n161 = Subtract(x="duration", y=w452) -> (x-y=w451:dbl)
              n162 = To Word Integer(number=w451) -> (16bit integer=→"contdown":i16)
              n163 = xnode "Read/Write Control"("FPGA VI Reference In"=w459, "error in"=w469, "Loop Period (ticks)"=w474) -> ("FPGA VI Reference Out"=w473:refnum<k20>, "error out"=w472:errorcluster, "FIFO Full?"=w449:bool)
              "FIFO full?" <- w449
              n164 = Greater Or Equal?(x=w452, y="duration") -> (x >= y?=w456:bool)
              n165 = xnode "Invoke Method"("FPGA VI Reference In"=w473, "error in"=w472, "Number of Elements"=u32 5000, "Timeout (ms)"=-1) -> ("FPGA VI Reference Out"=w457:refnum<k20>, "error out"=w458:errorcluster, "Data"=w468:i16[])  [unwired: 1 out]
              n166 = To Double Precision Float(number=w468) -> (double precision float=w447:dbl[])
              n167 = Multiply(x=w447, y=0.004883) -> (x*y=w444:dbl[])
              "Voltage" <- w444
              n168 = case shown="\"curva1\"" "curvas" {
                tunnel: w444 -> [w478 w482 _]
                tunnel: [w479 w481 dbl[] []] -> w445
                frame "curva5", Default {
                  n169 = expression code="-1.8491+(7.5461+1.891)/(1+exp((0.860921*ln(x/0.592216))))"(w478) -> (w479:dbl[])
                  n170 = property on="Current" class="Arr (strict)"("Visible"=TRUE) -> ()  [unwired: 2 in, 2 out]
                }
                frame "curva1" {
                  n171 = expression code="exp(-3.7042+1.03111*x)"(w482) -> (w481:dbl[])
                  n172 = property on="Current" class="Arr (strict)"("Visible"=TRUE) -> ()  [unwired: 2 in, 2 out]
                }
                frame "meas" {
                  n173 = property on="Current" class="Arr (strict)"("Visible"=FALSE) -> ()  [unwired: 2 in, 2 out]
                }
              }
              "Current" <- w445
              n174 = xnode "Read/Write Control"("FPGA VI Reference In"=w457, "error in"=w458, "Stop Button"=w456) -> ("FPGA VI Reference Out"=w454:refnum<k20>, "error out"=w455:errorcluster)
              n175 = Build Array (concatenate)(w452, w444) -> (w462:dbl[])
              n176 = Build Array (concatenate)(w461, w462) -> (w460:dbl[][])
              n177 = Compound Arithmetic op=OR(w449, w456, w455, "Stop Button") -> (w471:bool)
            }
          }
        }
        n178 = xnode "Invoke Method"("FPGA VI Reference In"=w435, "error in"=w434) -> ("FPGA VI Reference Out"=w424:refnum<k20>, "error out"=w423:errorcluster)
        n179 = Bundle By Name(cluster=w430, "frequency"=w412, "data"=w429) -> (w428:T2)
        n180 = Select(t=w416, s="save", f=w414) -> (s? t:f=w413:T3[])
        n181 = xnode "Close FPGA VI Reference"("FPGA VI Reference In"=w424, "error in"=w423) -> ("error out"=w422:errorcluster)
      }
      frame "save data" {
        w493 = T3[] [enum."idle"] items=["idle", "lock", "set", "reset", "get data", "save data"]
        n182 = Unbundle By Name(w492) -> ("data"=w486:dbl[][])
        n183 = call "txt.vi"("file name"="file name", "array"=w486, "error in"=w485) -> ("output cluster"=w489:T4, "error out"=w490:errorcluster)  [unwired: 9 in, 2 out]
        n184 = Unbundle(w489) -> ("mean"=→"Mean":dbl, "standard deviation"=→"Standart Deviation":dbl)  [unwired: 1 out]
      }
    }
  }
